vi "Get (Boolean).vi"(8 "error in":errorcluster, 11 "Value in":refnum<class "Value.lvclass">) -> (0 "error out":errorcluster, 1 "Is Defined?":bool, 2 "Value":bool, 3 "Value out":refnum<class "Value.lvclass">)   [LabVIEW 2024, in "Electronic Datasheet.lvlib" / "Value.lvclass"]
uses:
  Value.lvclass
  Value.lvclass/Value.ctl
  Electronic Datasheet.lvlib
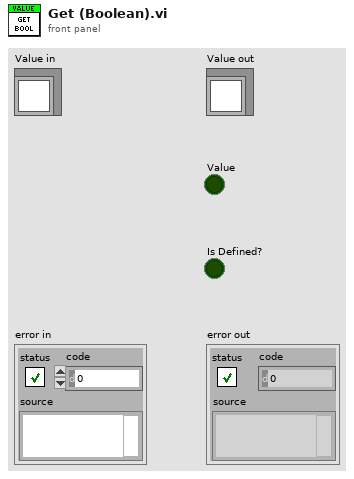
[diagram p1: front panel]
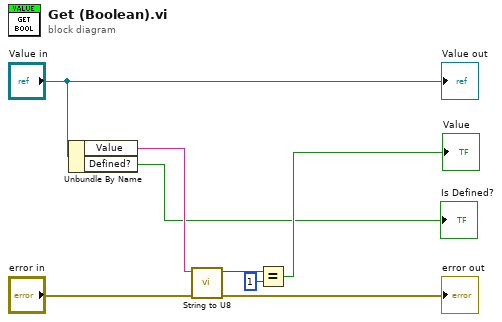
[diagram p0: block diagram]
diagram:
  n1 = Unbundle By Name("Value in") -> ("Value"=w7:string, "Defined?"=→"Is Defined?":bool)
  n2 = call "String to U8.vi"("error in"="error in", "String"=w7) -> ("error out"=→"error out":errorcluster, "U8"=w4:u8)  [unwired: 8 in]
  n3 = Equal?(x=w4, y=u8 1) -> (x = y?=→"Value":bool)
  "Value out" <- "Value in"
